vi "SetupPXI.vi"(10 "Experiment State":T1={"error"={"status"=FALSE, "code"=0, "source"=""}, "Digitizer DAQmx Tasks"={"TaskArray"=[]}, "Digitizer Settings"={"Channel Settings"=[], "Card Settings"=[]}, "Synchronization Settings"={"Synchronizer"="PXI1Slot2", "source terminal"="GlobalSoftwareTrigger"}, "Digitizer Data"=[], "Next Shot#"="0", "System Message"="", "User Shot Notes"="", "Timing Settings"={"Timing Card Settings"=[], "Timing Channel Settings"=[[{"Delay (s)"=2.559999942779541, "Pulse width (s)"=0.009999999776482582, "Active"=TRUE, "Channel Name"="Fiber 8", "counter"="PXI1Slot8/ctr7"}]]}, "Timing Tasks"={"TaskArray"=[]}, "Tree"="0"} {"Timing Settings"."Timing Channel Settings"."Pulse width (s)" format="%.3p"; "Timing Settings"."Timing Channel Settings"."Delay (s)" format="%.3p"; "Digitizer Settings"."Card Settings"."Global Edge Type" items=["Rising"=10280, "Falling"=10171]; "Digitizer Settings"."Card Settings"."Sample Rate" format="%#_3p"}) -> (2 "Experiment State":T1={"error"={"status"=FALSE, "code"=0, "source"=""}, "Digitizer DAQmx Tasks"={"TaskArray"=[]}, "Digitizer Settings"={"Channel Settings"=[], "Card Settings"=[]}, "Synchronization Settings"={"Synchronizer"="PXI1Slot2", "source terminal"="GlobalSoftwareTrigger"}, "Digitizer Data"=[], "Next Shot#"="0", "System Message"="", "User Shot Notes"="", "Timing Settings"={"Timing Card Settings"=[], "Timing Channel Settings"=[[{"Delay (s)"=2.559999942779541, "Pulse width (s)"=0.009999999776482582, "Active"=TRUE, "Channel Name"="Fiber 8", "counter"="PXI1Slot8/ctr7"}]]}, "Timing Tasks"={"TaskArray"=[]}, "Tree"="0"} {"Timing Settings"."Timing Channel Settings"."Pulse width (s)" format="%.3p"; "Timing Settings"."Timing Channel Settings"."Delay (s)" format="%.3p"; "Digitizer Settings"."Card Settings"."Global Edge Type" items=["Rising"=10280, "Falling"=10171]; "Digitizer Settings"."Card Settings"."Sample Rate" format="%#_3p"})   [LabVIEW 2013]
uses:
  Controls/ExperimentStateCluster.ctl
  Controls/DigitizerSettingsChannelSettings.ctl
  Controls/DigitizerSettingsCardSettingsArray.ctl
  Controls/DigitizerSettingsCardSettings.ctl
  Controls/TimingCardSettings.ctl
  Controls/TimingChannelSettings.ctl
  <instrlib>/niSync/niSync.llb/niSync Initialize (IVI).vi
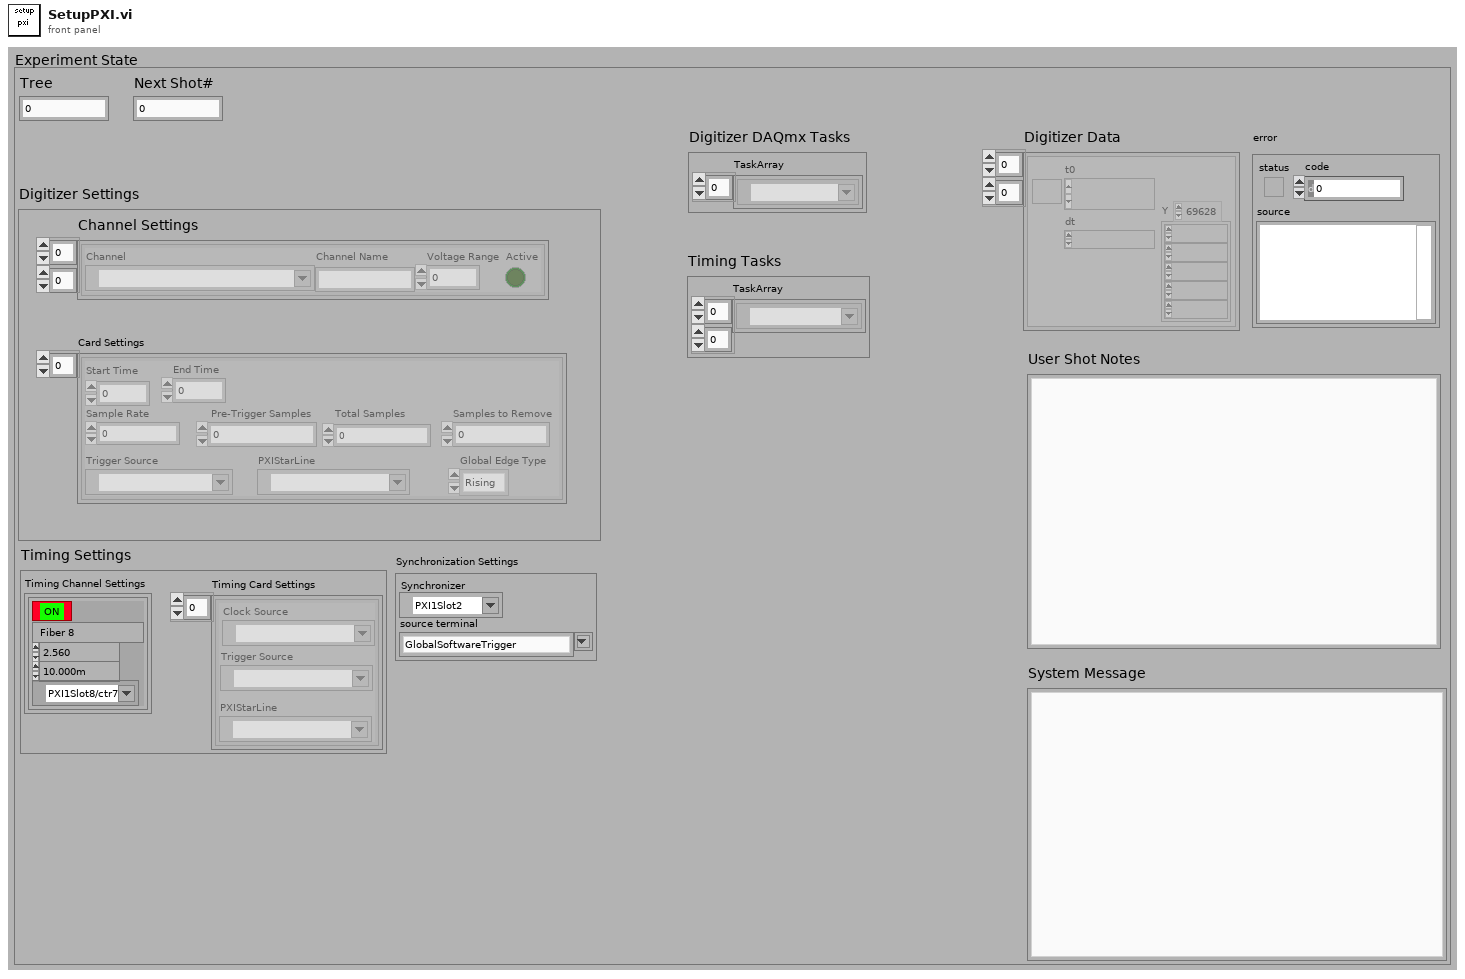
[diagram p1: front panel]
types:
  T1 = typedef "ExperimentStateCluster.ctl" = cluster{"error":errorcluster, "Digitizer DAQmx Tasks":cluster{"TaskArray":refnum<k21>[]}, "Digitizer Settings":cluster{"Channel Settings":T2[][], "Card Settings":T3}, "Synchronization Settings":cluster{"Synchronizer":refnum<k15>, "source terminal":string}, "Digitizer Data":waveform(dbl)[][], "Next Shot#":string, "System Message":string, "User Shot Notes":string, "Timing Settings":cluster{"Timing Card Settings":T5[], "Timing Channel Settings":T6[][]}, "Timing Tasks":cluster{"TaskArray":refnum<k21>[][]}, "Tree":string}
  T2 = typedef "DigitizerSettingsChannelSettings.ctl" = cluster{"Channel":tag, "Channel Name":string, "Voltage Range":dbl, "Active":bool}
  T3 = typedef "DigitizerSettingsCardSettingsArray.ctl" = T4[]
  T4 = typedef "DigitizerSettingsCardSettings.ctl" = cluster{"Start Time":dbl, "End Time":dbl, "Sample Rate":dbl, " Pre-Trigger Samples":u32, "Total Samples":i32, "Samples to Remove":u32, "Trigger Source":tag, "Global Edge Type":i32, "PXIStarLine":tag}
  T5 = typedef "TimingCardSettings.ctl" = cluster{"Trigger Source":tag, "Clock Source":tag, "PXIStarLine":tag}
  T6 = typedef "TimingChannelSettings.ctl" = cluster{"Delay (s)":dbl, "Pulse width (s)":dbl, "Active":bool, "Channel Name":string, "counter":tag}
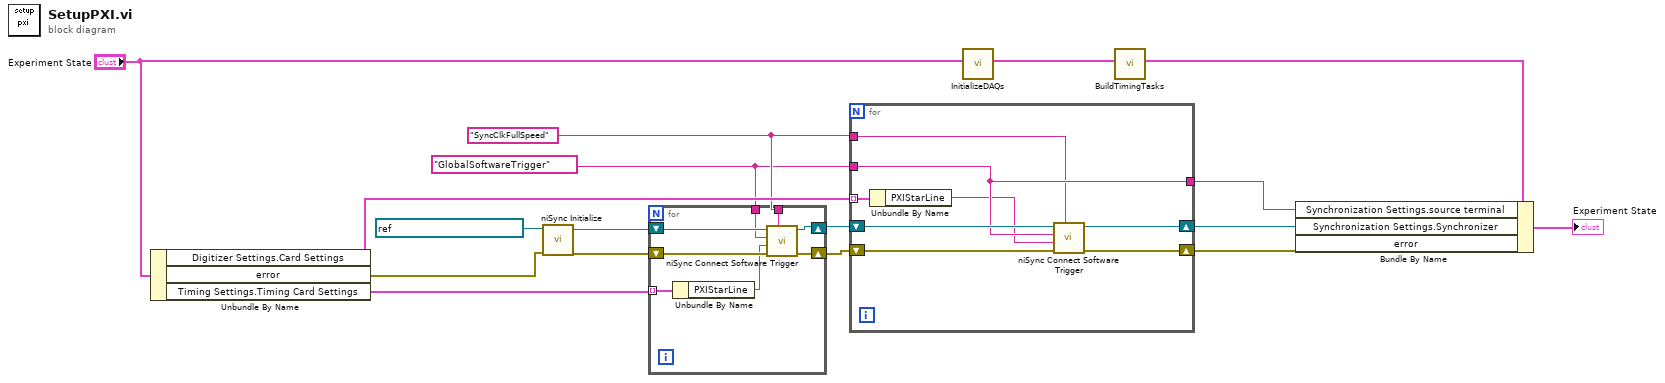
[diagram p0: block diagram]
diagram:
  w6 = "SyncClkFullSpeed" ("synchronization clock")
  w5 = "GlobalSoftwareTrigger" ("source terminal")
  n1 = Unbundle By Name("Experiment State") -> ("Digitizer Settings.Card Settings"=w7:T3, "error"=w15:errorcluster, "Timing Settings.Timing Card Settings"=w4:T5[])
  n2 = call-poly <instrlib>:"niSync Initialize.vi"("error in (no error)"=w15, "resource name"=refnum<k15> "Sync") -> ("error out"=w8:errorcluster, "instrument handle out"=w9:refnum<k15>)  [unwired: 1 in, 7 out]
  n3 = for {
    tunnel: w6 -> [w23]
    tunnel: w5 -> [w22]
    tunnel: w4 -> [w21] mode=indexing
    shift-right: [w19] -> w3
    shift-left: w8 -> [w24]
    shift-right: [w18] -> w2
    shift-left: w9 -> [w25]
    n4 = Unbundle By Name(w21) -> ("PXIStarLine"=w20:tag)
    n5 = call <instrlib>:"niSync Connect Software Trigger.vi"("synchronization clock"=w23, "error in (no error)"=w24, "destination terminal"=w20, "source terminal"=w22, "instrument handle"=w25) -> ("error out"=w19:errorcluster, "instrument handle out"=w18:refnum<k15>)  [unwired: 2 in, 3 out]
  }
  n6 = for {
    tunnel: w7 -> [w27] mode=indexing
    shift-right: [w32] -> w13
    shift-left: w2 -> [w33]
    shift-right: [w30] -> w14
    shift-left: w3 -> [w31]
    tunnel: [w29] -> w12
    tunnel: w5 -> [w29]
    tunnel: w6 -> [w28]
    n7 = Unbundle By Name(w27) -> ("PXIStarLine"=w26:tag)
    n8 = call <instrlib>:"niSync Connect Software Trigger.vi"("synchronization clock"=w28, "error in (no error)"=w31, "destination terminal"=w26, "source terminal"=w29, "instrument handle"=w33) -> ("error out"=w30:errorcluster, "instrument handle out"=w32:refnum<k15>)  [unwired: 2 in, 3 out]
  }
  n9 = call "InitializeDAQs.vi"("Experiment State"="Experiment State") -> ("Experiment State"=w16:T1)  [unwired: 1 in, 9 out]
  n10 = call "BuildTimingTasks.vi"("Experiment State"=w16) -> ("Experiment State"=w1:T1)  [unwired: 1 in, 9 out]
  n11 = Bundle By Name(cluster=w1, "Synchronization Settings.source terminal"=w12, "Synchronization Settings.Synchronizer"=w13, "error"=w14) -> (→"Experiment State":T1)
